vi "failure dialog.vi"(5 "friendly":bool=TRUE, 7 "delay":dbl=15.0 format="%#_13g", 9 "failure":T2 {"code" format="%.0x"}) -> ()   [LabVIEW 2013]
uses:
  failure.ctl
  dialog tree/Failures_VariantTree__VP.lvclass
  dialog tree/TreeSettings.ctl
  dialog tree/Browse Variant_SetRef.vi
  failure.lvlib
panel:
  in  "commands":T1
  out "image":picture
  in  "probe":string[](tree)
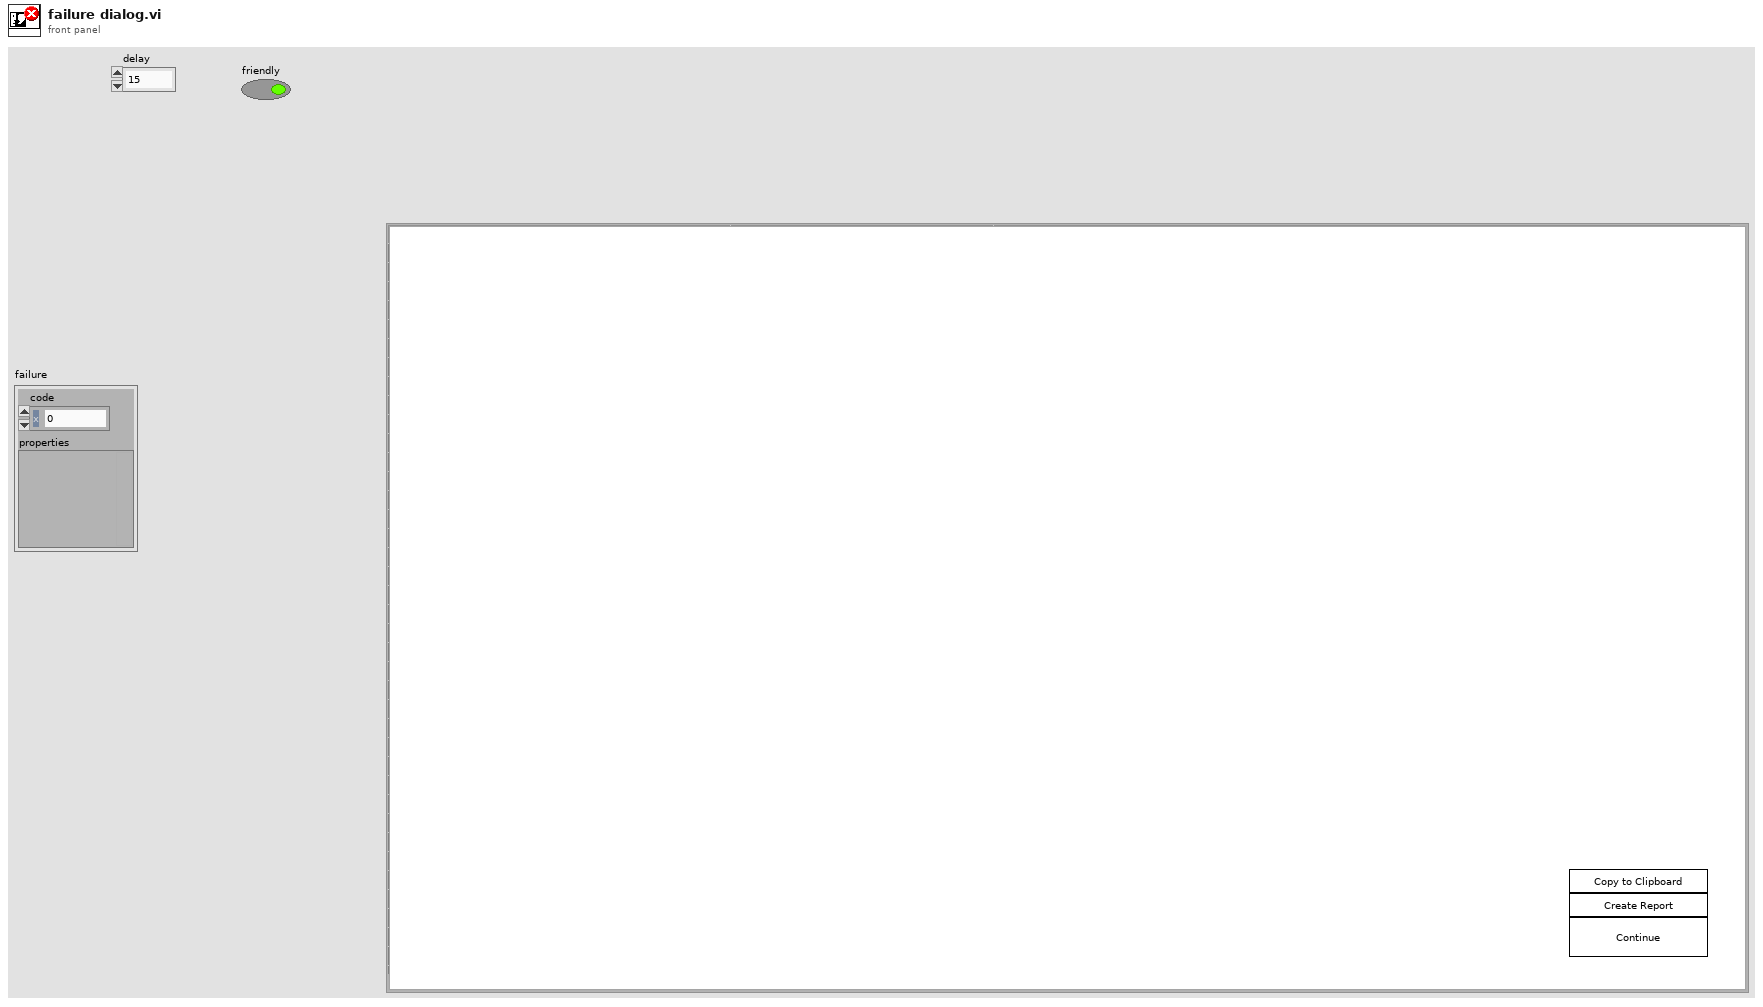
[diagram p1: front panel]
types:
  T1 = cluster{"copy to clipboard":bool, "create report":bool, "OK":bool}
  T2 = typedef "failure.lvlib/failure.ctl" = cluster{"code":i32, "properties":variant}
  T3 = typedef "Failures_VariantTree__VP.lvclass/TreeSettings.ctl" = cluster{"Traverse":bool, "Colorize":bool}
  T4 = enum32{"Invalid", "Standard", "Closed", "Hidden", "Minimized", "Maximized"}
  T5 = enum8{"Enabled", "Disabled", "Disabled and Grayed Out"}
  T6 = enum16{"open", "replace", "create", "open or create", "replace or create", "replace or create with confirmation"}
  T7 = cluster{"horizontal":enum16{"left", "center", "right"}, "vertical":enum16{"top", "center", "bottom"}}
  T8 = cluster{"left":i16, "top":i16, "right":i16, "bottom":i16}
  T9 = cluster{"Font Name:":string, "Size":i16, "Strikeout?":bool, "Italic?":bool, "Underline?":bool, "Outline?":bool, "Shadow?":bool, "Bold?":bool}
  T10 = enum16{"User-specified Font", "Application Font", "System Font", "Dialog Font"}
  T11 = typedef "LVBoundsTypeDef.ctl" = cluster{"Width":u32, "Height":u32}
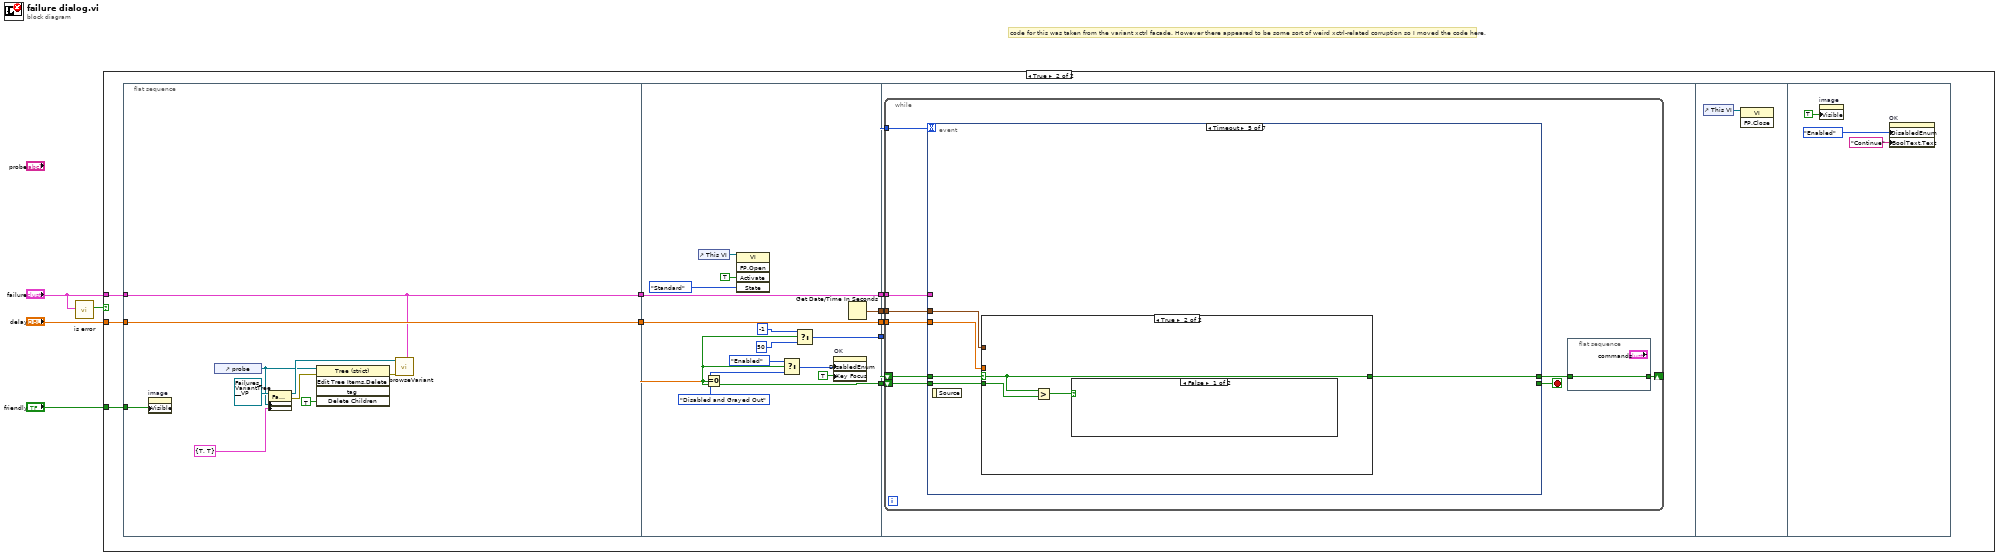
[diagram p0: block diagram]
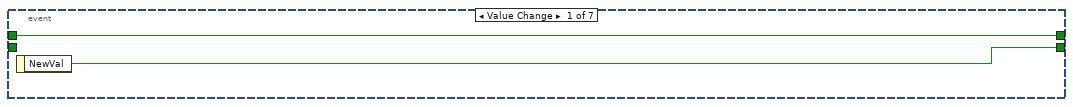
[diagram p3: hidden frame]
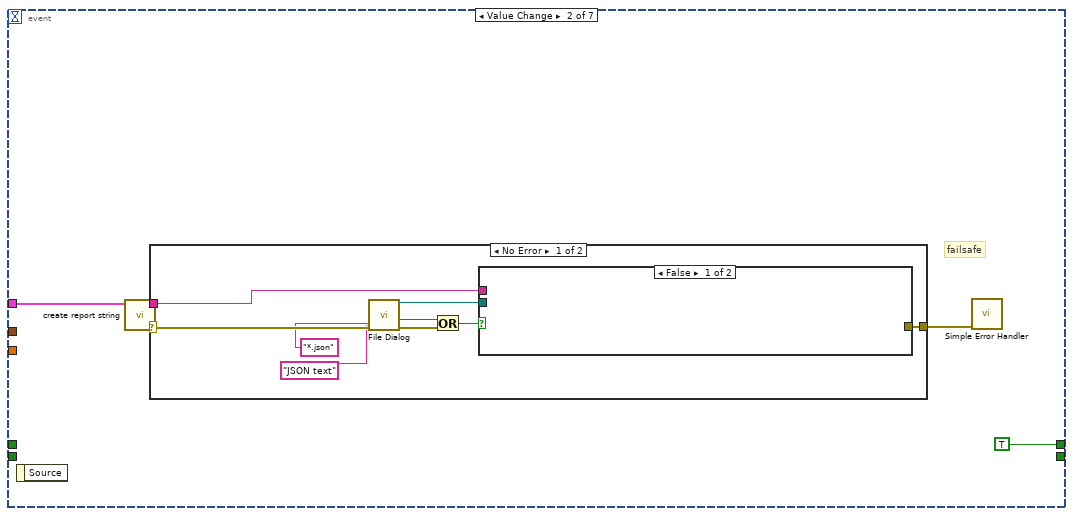
[diagram p4: hidden frame]
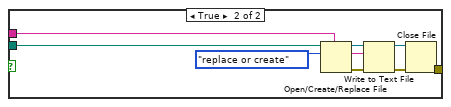
[diagram p5: hidden frame]
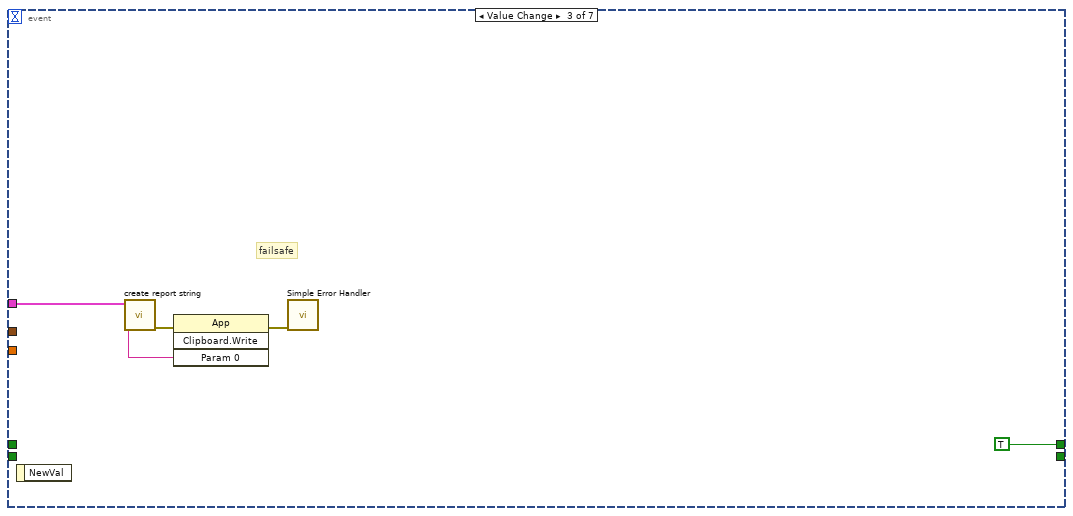
[diagram p7: hidden frame]
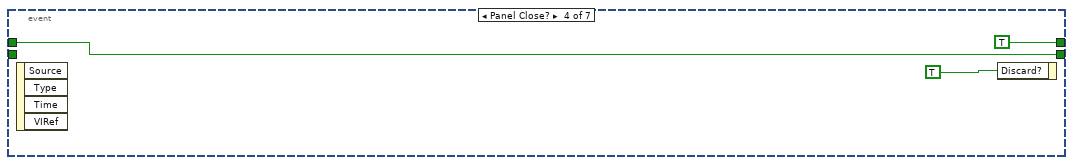
[diagram p8: hidden frame]
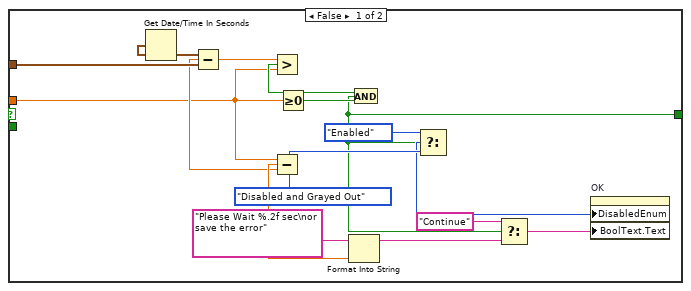
[diagram p9: hidden frame]
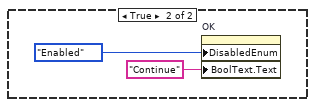
[diagram p10: hidden frame]
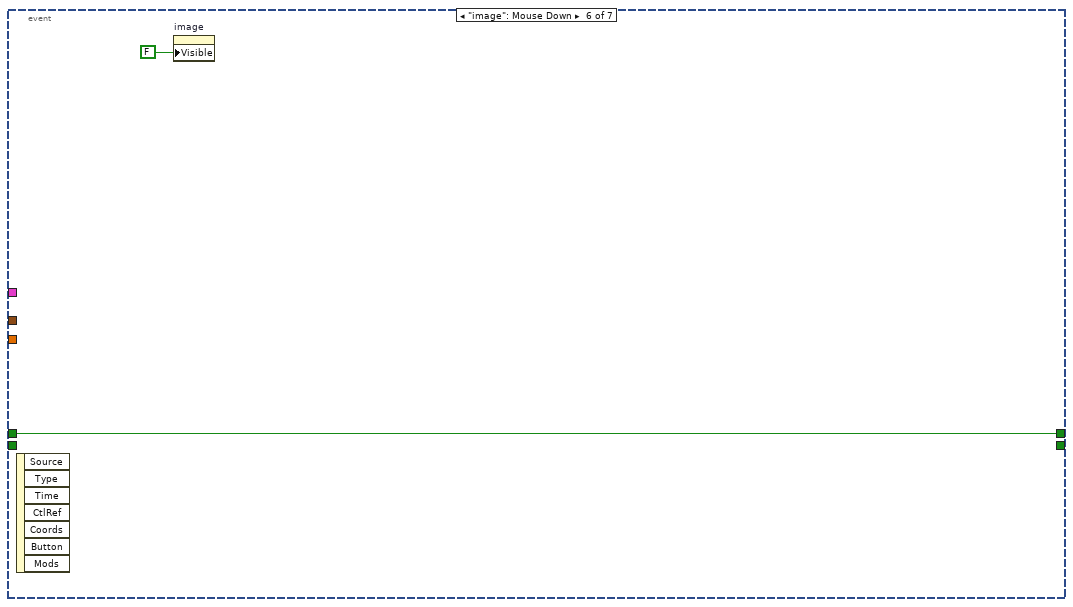
[diagram p11: hidden frame]
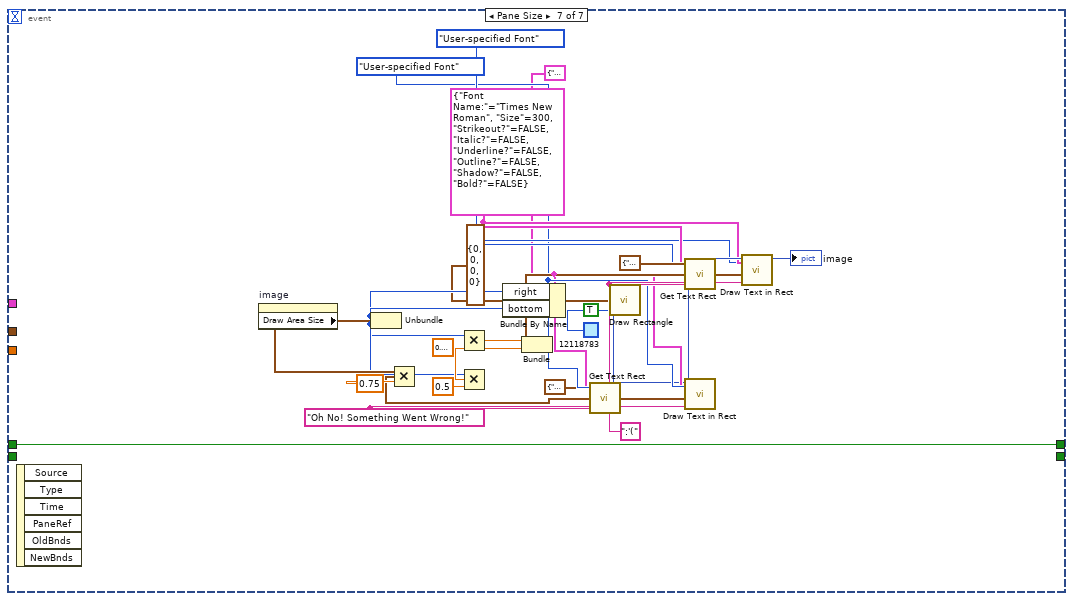
[diagram p12: hidden frame]
diagram:
  # "code for this was taken from the variant xctrl facade. However there appeared to be some sort of weird xctrl-related corruption so I moved the code here."
  n1 = call "is error.vi"("failure"="failure") -> ("error!"=w2:bool)  [unwired: 10 in]
  n2 = case shown="True" w2 {
    tunnel: "friendly" -> [_ w7]
    tunnel: "delay" -> [_ w6]
    tunnel: "failure" -> [_ w5]
    frame False {
    }
    frame True {
      n3 = flat-sequence {
        tunnel: [w23] -> w14
        tunnel: w7 -> [w22]
        tunnel: [w24] -> w13
        tunnel: w6 -> [w24]
        tunnel: w5 -> [w23]
        tunnel: w14 -> [w25]
        tunnel: [w25] -> w12
        tunnel: [w33] -> w11
        tunnel: [w32] -> w10
        tunnel: [w31] -> w9
        tunnel: [w30] -> w8
        tunnel: w13 -> [w30]
        tunnel: w12 -> [w43]
        tunnel: w11 -> [w42]
        tunnel: w10 -> [w41]
        tunnel: w9 -> [w39]
        tunnel: w8 -> [w40]
        frame #0 {
          n4 = property on="image" class="Pict"("Visible"=w22) -> ()  [unwired: 2 in, 2 out]
          n5 = control-ref of="probe"() -> (w17:refnum<vi>)
          n6 = property class="Failures_VariantTree__VP.lvclas"(reference=refnum<class "Failures_VariantTree__VP.lvclass"> refnum ("Dummy Class.lvclass"), "Reference"=w17, "SetOptions"=T3 {"Traverse"=TRUE, "Colorize"=TRUE} ("TreeSettings")) -> (reference out=w18:refnum<class "Failures_VariantTree__VP.lvclass">, error out=w16:errorcluster)  [unwired: 1 in]
          n7 = invoke class="Tree (strict)" method="Edit Tree Items.Delete"(reference=w17, error in=w16, "Delete Children"=TRUE ("Delete Children?")) -> (error out=w19:errorcluster)  [unwired: 2 in, 4 out]
          n8 = call-dynamic "browseVariant.vi"("Variant"=w23, "error in (no error)"=w19, "VariantProbe.lvclass in"=w18) -> ()  [unwired: 5 in, 2 out]
        }
        frame #1 {
          n9 = control-ref of="This VI"() -> (w29:refnum<vi>)
          n10 = Equal To 0?(x=w30) -> (x = 0?=w31:bool)
          n11 = invoke class="VI" method="FP.Open"(reference=w29, "Activate"=TRUE ("Activate?"), "State"=T4."Standard") -> ()  [unwired: 2 in, 5 out]
          n12 = Select(t=T5."Enabled" ("Disabled"), s=w31, f=T5."Disabled and Grayed Out" ("Disabled")) -> (s? t:f=w37:T5)
          n13 = Select(t=-1, s=w31, f=50) -> (s? t:f=w33:i32)
          n14 = property on="OK" class="Bool"("DisabledEnum"=w37, "Key Focus"=TRUE) -> ()  [unwired: 2 in, 2 out]
          n15 = Get Date/Time In Seconds() -> (seconds since 1Jan1904=w32:timestamp)
        }
        frame #2 {
          n16 = while {
            tunnel: w43 -> [w51]
            tunnel: w41 -> [w49]
            shift-right: [w45] -> _
            shift-left: w39 -> [w48]
            tunnel: w40 -> [w47]
            tunnel: w42 -> [w50]
            shift-left: w39 -> [w46]
            stop <- w52 stop-if-true
            n17 = event shown="[4] Timeout" {
              selector: _ -> [_ _ _ _ _ _ _]
              dyn-events: _ -> [_ _ _ _ _ _ _]
              timeout: w50 -> [_ _ _ _ _ _ _]
              tunnel: [w54 _ _ w85 _ _ _] -> w52
              tunnel: w51 -> [_ w58 w81 _ _ _ _]
              tunnel: w49 -> [_ _ _ _ w91 _ _]
              tunnel: w48 -> [w55 _ _ w85 w88 w113 w141]
              tunnel: [w55 TRUE TRUE TRUE w89 w113 w141] -> w44
              tunnel: w47 -> [_ _ _ _ w90 _ _]
              tunnel: w46 -> [_ _ _ _ w87 _ _]
              event "commands.OK": Value Change {
                n18 = event-data() -> ("NewVal"=w54:bool)  [unwired: 1 in]
              }
              event "commands.create report": Value Change {
                # "failsafe"
                n19 = event-data() -> ()  [unwired: 1 in, 1 out]
                n20 = call "create report string.vi"("failure"=w58) -> ("error out"=w57:errorcluster, "report string"=w56:string)  [unwired: 9 in]
                n21 = case shown="No Error" w57 {
                  selector: w57 -> [w69 w78]
                  tunnel: w56 -> [w63 _]
                  tunnel: [w61 w78] -> w59
                  frame No Error {
                    n22 = call "File Dialog"("error in"=w69, "pattern (all files)"="*.json", "pattern label"="JSON text") -> ("selected path"=w62:path, "cancelled"=w66:bool, "error out"=w64:errorcluster)  [unwired: 9 in, 1 out]
                    n23 = Or(x=w66, y=w64) -> (x .or. y?=w65:bool)
                    n24 = case shown="False" w65 {
                      tunnel: w63 -> [_ w73]
                      tunnel: w62 -> [_ w72]
                      tunnel: [_ w70] -> w61
                      frame False {
                      }
                      frame True {
                        n25 = Open/Create/Replace File(file path (use dialog)=w72, operation (0:open)=T6."replace or create") -> (refnum out=w77:refnum<file>, error out=w74:errorcluster)  [unwired: 4 in, 1 out]
                        n26 = Write to Text File(file (use dialog)=w77, text=w73, error in=w74) -> (refnum out=w76:refnum<file>, error out=w75:errorcluster)  [unwired: 1 in, 1 out]
                        n27 = Close File(refnum=w76, error in=w75) -> (error out=w70:errorcluster)  [unwired: 1 out]
                      }
                    }
                  }
                  frame Error {
                  }
                }
                n28 = call <vilib>:"Simple Error Handler.vi"("error in (no error)"=w59) -> ()  [unwired: 4 in, 5 out]
              }
              event "commands.copy to clipboard": Value Change {
                # "failsafe"
                n29 = event-data() -> ()  [unwired: 1 in, 1 out]
                n30 = call "create report string.vi"("failure"=w81) -> ("error out"=w83:errorcluster, "report string"=w82:string)  [unwired: 9 in]
                n31 = invoke class="App" method="Clipboard.Write"(error in=w83, "Param 0"=w82) -> (error out=w80:errorcluster)  [unwired: 2 in, 3 out]
                n32 = call <vilib>:"Simple Error Handler.vi"("error in (no error)"=w80) -> ()  [unwired: 4 in, 5 out]
              }
              event Panel Close? {
                n33 = event-data() -> ()  [unwired: 1 in, 4 out]
                n34 = event-data("Discard?"=TRUE) -> ()  [unwired: 1 in, 1 out]
              }
              event Timeout {
                n35 = event-data() -> ()  [unwired: 1 in, 1 out]
                n36 = case shown="True" w88 {
                  selector: w88 -> [_ w109]
                  tunnel: w91 -> [w105 _]
                  tunnel: w90 -> [w96 _]
                  tunnel: [w92 w109] -> w89
                  tunnel: w87 -> [_ w108]
                  frame False {
                    n37 = Get Date/Time In Seconds() -> (seconds since 1Jan1904=w106:timestamp)
                    n38 = Subtract(x=w106, y=w105) -> (x-y=w97:dbl)
                    n39 = Greater?(x=w97, y=w96) -> (0:w100:bool)
                    n40 = Subtract(x=w96, y=w97) -> (x-y=w98:dbl)
                    n41 = Greater Or Equal To 0?(x=w96) -> (x >= 0?=w101:bool)
                    n42 = Format Into String(format string="Please Wait %.2f sec\nor save the error", w98) -> (resulting string=w93:string)  [unwired: 2 in, 1 out]
                    n43 = And(x=w100, y=w101) -> (x .and. y?=w92:bool)
                    n44 = Select(t=T5."Enabled" ("Disabled"), s=w92, f=T5."Disabled and Grayed Out" ("Disabled")) -> (s? t:f=w103:T5)
                    n45 = Select(t="Continue" ("Boolean Text.Text"), s=w92, f=w93) -> (s? t:f=w94:string)
                    n46 = property on="OK" class="Bool"("DisabledEnum"=w103, "BoolText.Text"=w94) -> ()  [unwired: 2 in, 2 out]
                  }
                  frame True {
                    n47 = Greater?(x=w109, y=w108) -> (0:w107:bool)
                    n48 = case shown="False" w107 {
                      frame False {
                      }
                      frame True {
                        n49 = property on="OK" class="Bool"("DisabledEnum"=T5."Enabled" ("Disabled"), "BoolText.Text"="Continue" ("Boolean Text.Text")) -> ()  [unwired: 2 in, 2 out]
                      }
                    }
                  }
                }
              }
              event "image": Mouse Down {
                n50 = event-data() -> ()  [unwired: 1 in, 7 out]
                n51 = property on="image" class="Pict"("Visible"=FALSE) -> ()  [unwired: 2 in, 2 out]
              }
              event Pane Size {
                w127 = T9 {"Font Name:"="Times New Roman", "Size"=300, "Strikeout?"=FALSE, "Italic?"=FALSE, "Underline?"=FALSE, "Outline?"=FALSE, "Shadow?"=FALSE, "Bold?"=FALSE} ("[user-specified font]")
                w126 = T10."User-specified Font" ("desired font(Application)")
                w129 = ":'(" ("text")
                w124 = T9 {"Font Name:"="Times New Roman", "Size"=25, "Strikeout?"=FALSE, "Italic?"=TRUE, "Underline?"=FALSE, "Outline?"=FALSE, "Shadow?"=FALSE, "Bold?"=FALSE} ("[user-specified font]")
                w125 = T10."User-specified Font" ("desired font(Application)")
                w120 = "Oh No! Something Went Wrong!" ("text")
                n52 = event-data() -> ()  [unwired: 1 in, 6 out]
                n53 = property on="image" class="Pict"() -> ("Draw Area Size"=w139:T11)  [unwired: 2 in, 2 out]
                n54 = Unbundle(w139) -> ("Width"=w132:u32, "Height"=w134:u32)
                n55 = Multiply(x=w139, y=0.75) -> (x*y=w122:cluster{"Width":dbl, "Height":dbl})
                n56 = Multiply(x=w132, y=sgl 0.2) -> (x*y=w135:sgl)
                n57 = Multiply(x=w134, y=sgl 0.5) -> (x*y=w136:sgl)
                n58 = Bundle By Name(cluster=T8 {"left"=0, "top"=0, "right"=0, "bottom"=0} ("rect"), "right"=w132, "bottom"=w134) -> (w115:T8)
                n59 = Bundle(w135, w136) -> (w137:cluster{sgl, sgl})  [unwired: 1 in]
                n60 = call <vilib>:"Get Text Rect.vi"("alignment(left, top)"=T7 {"horizontal"=enum."center", "vertical"=enum."center"}, "desired font(Application)"=w125, "origin(0,0)"=w122, "text"=w120, "[user-specified font]"=w124) -> ("rect"=w121:T8)  [unwired: 4 in]
                n61 = call <vilib>:"Draw Rectangle.vi"("rect"=w115, "fill?(F)"=TRUE, "color(black)"=u32 12118783) -> ("new picture"=w118:picture)  [unwired: 6 in]
                n62 = call <vilib>:"Get Text Rect.vi"("alignment(left, top)"=T7 {"horizontal"=enum."center", "vertical"=enum."center"}, "desired font(Application)"=w126, "origin(0,0)"=w137, "text"=w129, "[user-specified font]"=w127) -> ("rect"=w128:T8)  [unwired: 4 in]
                n63 = call <vilib>:"Draw Text in Rect.vi"("[user-specified font]"=w124, "desired font(Application)"=w125, "text"=w120, "rect"=w121, "picture"=w118) -> ("new picture"=w131:picture)  [unwired: 6 in]
                n64 = call <vilib>:"Draw Text in Rect.vi"("[user-specified font]"=w127, "desired font(Application)"=w126, "text"=w129, "rect"=w128, "picture"=w131) -> ("new picture"=→"image":picture)  [unwired: 6 in]
              }
            }
            n65 = flat-sequence {
              tunnel: [w53] -> w45
              tunnel: w44 -> [w53]
              frame #0 {
              }
            }
          }
        }
        frame #3 {
          n66 = control-ref of="This VI"() -> (w142:refnum<vi>)
          n67 = invoke class="VI" method="FP.Close"(reference=w142) -> ()  [unwired: 2 in, 3 out]
        }
        frame #4 {
          n68 = property on="image" class="Pict"("Visible"=TRUE) -> ()  [unwired: 2 in, 2 out]
          n69 = property on="OK" class="Bool"("DisabledEnum"=T5."Enabled" ("Disabled"), "BoolText.Text"="Continue" ("Boolean Text.Text")) -> ()  [unwired: 2 in, 2 out]
        }
      }
    }
  }
